vi "Compass.vi"() -> ()   [LabVIEW 2014]
uses:
  <vilib>/Math Plots/2D Math Plots/2D Compass/2D Compass Datatype/2D Compass Datatype.lvclass
  <vilib>/Math Plots/2D Math Plots/2D Compass/2D Compass Datatype/Public/Plot Helper (Vector).vi
panel:
  out "Gyro":dbl(knob) scale=0.0..360.0
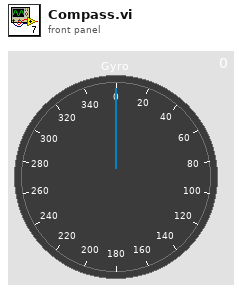
[diagram p1: front panel]
types:
  T1 = cluster{"maximum":dbl, "minimum":dbl, "clip to min":bool, "log?(F)":bool, "grid color":u32, "plot color":u32, "fmt and prec":cluster{"format":enum8{"Decimal", "Scientific", "Engineering", "Binary", "Octal", "Hex"}, "precision":u8}, "visible section":u16}
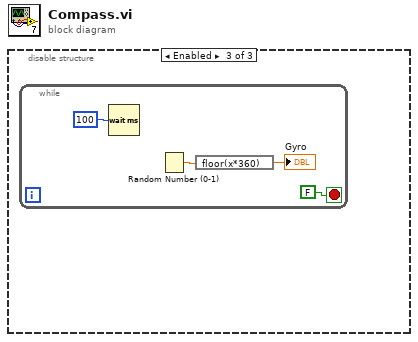
[diagram p0: block diagram]
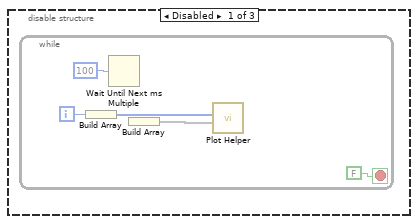
[diagram p2: hidden frame]
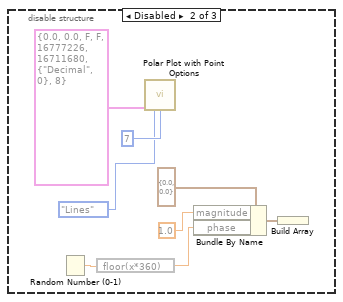
[diagram p3: hidden frame]
diagram:
  n1 = disable-structure shown="Enabled" {
    frame Disabled {
      n2 = while {
        i -> [w1]
        stop <- FALSE stop-if-true
        n3 = Build Array(w1) -> (w3:i32[])
        n4 = Wait Until Next ms Multiple(millisecond multiple=u32 100) -> ()  [unwired: 1 out]
        n5 = Build Array() -> (w4:void[], w5:dbl)
        n6 = call-poly <vilib>:"Plot Helper.vi"("radius vector"=w4, "theta vector"=w3) -> ("2D Plot Class Obj Array out"=w7:refnum<class "2D Plot Datatype.lvclass">[])  [unwired: 2 in, 7 out]
      }
    }
    frame Disabled {
      n7 = Random Number (0-1)() -> (number: 0 to 1=w13:dbl)
      n8 = expression code="floor(x*360)"(w13) -> (w10:dbl)
      n9 = call <vilib>:"Polar Plot with Point Options.vi"("polar attributes"=T1 {"maximum"=0.0, "minimum"=0.0, "clip to min"=FALSE, "log?(F)"=FALSE, "grid color"=16777226, "plot color"=16711680, "fmt and prec"={"format"=enum."Decimal", "precision"=0}, "visible section"=8}, "Lines/Points"=enum16{"Lines", "Points"}."Lines", "Size"=u16 7) -> ("new picture"=w17:picture, "data array [mag, phase (deg)]"=w8:cluster{"magnitude":dbl, "phase":dbl}[], "dimensions (w,h)"=w18:cluster{"width":i16, "height":i16})  [unwired: 10 in]
      n10 = Bundle By Name(cluster=cluster{"magnitude":dbl, "phase":dbl} {"magnitude"=0.0, "phase"=0.0}, "magnitude"=1.0, "phase"=w10) -> (w11:cluster{"magnitude":dbl, "phase":dbl})
      n11 = Build Array(w11) -> ()  [unwired: 1 out]
    }
    frame Enabled {
      n12 = while {
        stop <- FALSE stop-if-true
        n13 = Wait (ms)(milliseconds to wait=u32 100) -> ()  [unwired: 1 out]
        n14 = Random Number (0-1)() -> (number: 0 to 1=w21:dbl)
        n15 = expression code="floor(x*360)"(w21) -> (→"Gyro":dbl)
      }
    }
  }
